vi "Drive Motor TXRX.vi"(0 "Error In":errorcluster, 1 "Drive Motor Handle In":T2, 2 "Open Loop Current Flag":bool, 3 "Tasking Period":dbl, 4 "RPM Control (rad/s)":dbl, 5 "Controller Data In":refnum<data-value>, 6 "Speed Control (m/s)":dbl, 7 "?":T3={"Accelerometer Bias"={"X (m/s)"=0.0, "Y (m/s)"=0.0, "Z (m/s)"=0.0}, "Gyroscope Bias"={"X (m/s)"=0.0, "Y (m/s)"=0.0, "Z (m/s)"=0.0}, "Steering Motor Gear Ratio"=611.0, "Steering Pully Gear Ratio"=1.0, "Steering Encoder CPR"=500.0, "Steering Motor Max RPM"=4000.0, "Wheelbase (m)"=1.12, "Fork Angle (rad)"=1.3, "Balancing Controller"={"Kp (/s)"=0.0, "Kd (1)"=0.0}, "Max Allowed Steering Angle (rad)"=0.7, "Task Periods"={"Emergency Stop (us)"=0, "IMU (us)"=0, "Steering Motor Encoder (us)"=0, "State Estimator (us)"=0, "Balancing Controller (us)"=0, "GNSS (us)"=0, "Logging (us)"=0, "Drive Motor (us)"=0, "Visualization (us)"=50000}, "Drive Motor Gear Ratio"=0.7, "lr"=0.0, "lf"=0.0, "lambda"=0.0, "k1"=0.0, "k2"=0.0, "e1_max"=0.0, "Ad_t"=0.0, "Bd_t"=0.0, "C_t"=0.0, "D_t"=0.0, "Wheel radius"=0.311}, 10 "No Kf":bool, 11 "Ki":dbl, 12 "RPM / Speed":bool, 13 "Kp":dbl, 16 "Open Loop Current":dbl min=0.0, 17 "Kf":dbl min=0.0) -> (14 "Error Out":errorcluster, 15 "Drive Motor Handle Out":T2, 18 "Drive Motor Data":T1, 19 "Controller Data Out":refnum<data-value>)   [LabVIEW 2021]
uses:
  Drive Motor Handle.ctl
  Configuration/Configuration.ctl
  Drive Motor Data.ctl
  Logging/Controller Data.ctl
  Steering Motor/Steering Motor Data.ctl
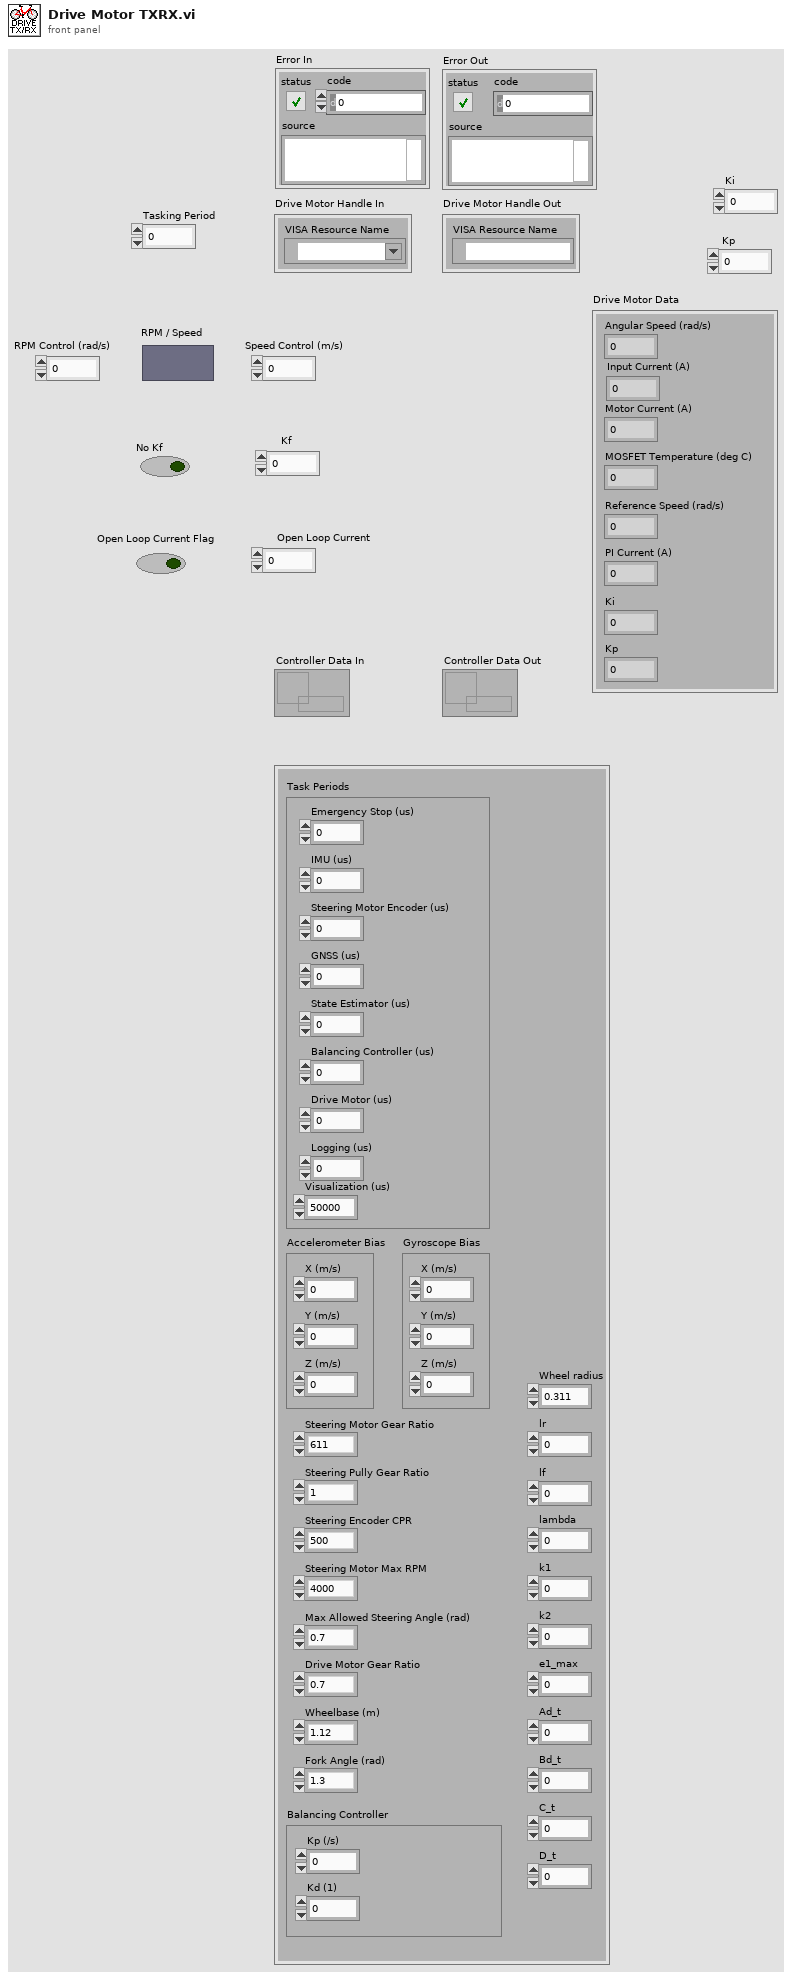
[diagram p1: front panel]
types:
  T1 = typedef "Drive Motor Data.ctl" = cluster{"Angular Speed (rad/s)":dbl, "Input Current (A)":dbl, "Motor Current (A)":dbl, "MOSFET Temperature (deg C)":dbl, "Reference Speed (rad/s)":dbl, "PI Current (A)":dbl, "Ki":dbl, "Kp":dbl}
  T2 = typedef "Drive Motor Handle.ctl" = cluster{"VISA Resource Name":refnum<visa-resource-name>}
  T3 = typedef "Configuration.ctl" = cluster{"Accelerometer Bias":cluster{"X (m/s)":dbl, "Y (m/s)":dbl, "Z (m/s)":dbl}, "Gyroscope Bias":cluster{"X (m/s)":dbl, "Y (m/s)":dbl, "Z (m/s)":dbl}, "Steering Motor Gear Ratio":dbl, "Steering Pully Gear Ratio":dbl, "Steering Encoder CPR":dbl, "Steering Motor Max RPM":dbl, "Wheelbase (m)":dbl, "Fork Angle (rad)":dbl, "Balancing Controller":cluster{"Kp (/s)":dbl, "Kd (1)":dbl}, "Max Allowed Steering Angle (rad)":dbl, "Task Periods":cluster{"Emergency Stop (us)":i64, "IMU (us)":i64, "Steering Motor Encoder (us)":i64, "State Estimator (us)":i64, "Balancing Controller (us)":i64, "GNSS (us)":i64, "Logging (us)":i64, "Drive Motor (us)":i64, "Visualization (us)":i64}, "Drive Motor Gear Ratio":dbl, "lr":dbl, "lf":dbl, "lambda":dbl, "k1":dbl, "k2":dbl, "e1_max":dbl, "Ad_t":dbl, "Bd_t":dbl, "C_t":dbl, "D_t":dbl, "Wheel radius":dbl}
  T4 = typedef "Controller Data.ctl" = cluster{"Drive Motor Data":T1, "Steering Motor Data":T5}
  T5 = typedef "Steering Motor Data.ctl" = cluster{"PWM":dbl, "Steering Angle Rate (rad/s)":dbl, "input balancing":dbl}
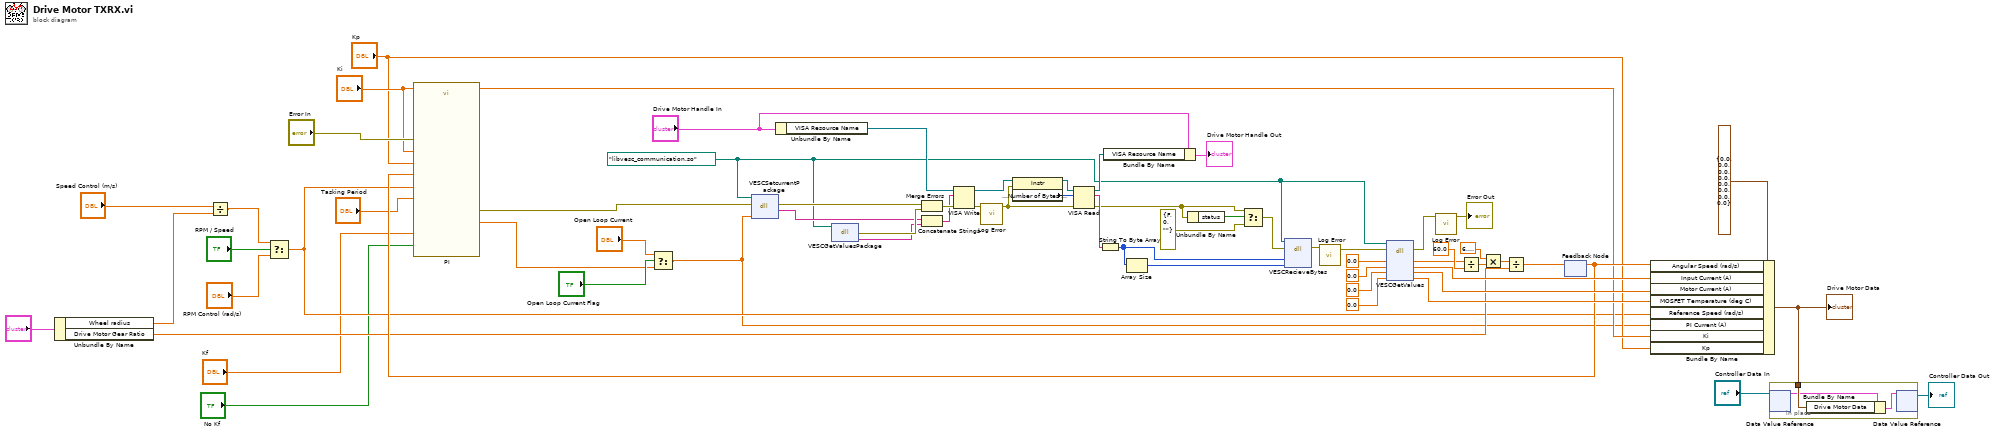
[diagram p0: block diagram]
diagram:
  w21 = path "libvesc_communication.so" ("path in")
  n1 = Unbundle By Name("?") -> ("Wheel radius"=w9:dbl, "Drive Motor Gear Ratio"=w8:dbl)
  n2 = Divide(x="Speed Control (m/s)", y=w9) -> (x/y=w14:dbl)
  n3 = Select(t=w14, s="RPM / Speed", f="RPM Control (rad/s)") -> (s? t:f=w7:dbl)
  n4 = Unbundle By Name("Drive Motor Handle In") -> ("VISA Resource Name"=w60:refnum<visa-resource-name>)
  n5 = dll-call lib="?" fn="VESCGetValuesPackage"(path in=w21) -> (error out=w59:errorcluster, "Package"=w25:string)  [unwired: 2 in, 1 out]
  n6 = feedback #1() -> (w18:dbl)  [unwired: 1 in]
  n7 = call "PI.vi"("Tasking Period"="Tasking Period", "Kp"="Kp", "Reference Speed (rad/s)"=w7, "Ki"="Ki", "Real Speed (rad/s)"=w18, "No Kf"="No Kf", "Kf"="Kf", "Error In"="Error In") -> ("PI Current (A)"=w2:dbl, "Error Out"=w17:errorcluster)  [unwired: 2 in]
  n8 = Select(t="Open Loop Current", s="Open Loop Current Flag", f=w2) -> (s? t:f=w1:dbl)
  n9 = dll-call lib="?" fn="VESCSetcurrentPackage"(path in=w21, error in=w17, "current"=w1) -> (error out=w22:errorcluster, "Package"=w23:string)  [unwired: 2 in, 1 out]
  n10 = Merge Errors(w22, w59) -> (w58:errorcluster)
  n11 = Concatenate Strings(w23, w25) -> (w24:string)
  n12 = VISA Write(VISA resource name=w60, write buffer=w24, error in (no error)=w58) -> (VISA resource name out=w57:refnum<visa-resource-name>, error out=w63:errorcluster)  [unwired: 1 out]
  n13 = call "Log Error.vi"("Error In"=w63) -> ("Error Out"=w45:errorcluster)  [unwired: 10 in]
  n14 = property class="Instr"(reference=w57, error in=w45) -> (reference out=w52:refnum<visa-resource-name>, "Serial Settings:Number of Bytes at Serial Port"=w55:u32)  [unwired: 1 out]
  n15 = VISA Read(VISA resource name=w52, byte count=w55, error in (no error)=w45) -> (VISA resource name out=w56:refnum<visa-resource-name>, read buffer=w54:string, error out=w53:errorcluster)  [unwired: 1 out]
  n16 = String To Byte Array(string=w54) -> (unsigned byte array=w50:u8[])
  n17 = Bundle By Name(cluster="Drive Motor Handle In", "VISA Resource Name"=w56) -> (→"Drive Motor Handle Out":T2)
  n18 = Array Size(array=w50) -> (size(s)=w51:i32)
  n19 = Unbundle By Name(w53) -> ("status"=w49:bool)
  n20 = Select(t=w53, s=w49, f=errorcluster {"status"=FALSE, "code"=0, "source"=""}) -> (s? t:f=w48:errorcluster)
  n21 = dll-call lib="?" fn="VESCRecieveBytes"(path in=w21, error in=w48, "bytes"=w50, "length"=w51) -> (error out=w46:errorcluster)  [unwired: 4 in, 1 out]
  n22 = call "Log Error.vi"("Error In"=w46) -> ("Error Out"=w26:errorcluster)  [unwired: 10 in]
  n23 = dll-call lib="?" fn="VESCGetValues"(path in=w21, error in=w26, "RPM"=0.0, "currentIn"=0.0, "currentMotor"=0.0 ("RPM"), "tempMOS"=0.0 ("currentIn")) -> (error out=w36:errorcluster, "RPM"=w34:dbl, "currentIn"=w33:dbl, "currentMotor"=w38:dbl, "tempMOS"=w27:dbl)  [unwired: 2 in, 1 out]
  n24 = call "Log Error.vi"("Error In"=w36) -> ("Error Out"=→"Error Out":errorcluster)  [unwired: 10 in]
  n25 = Divide(x=w34, y=60.0 ("x")) -> (x/y=w40:dbl)
  n26 = Multiply(x=6.283185307179586, y=w40) -> (x*y=w32:dbl)
  n27 = Divide(x=w32, y=w8) -> (x/y=w19:dbl)
  n28 = feedback-in #1(w19) -> ()
  n29 = Bundle By Name(cluster=T1 {"Angular Speed (rad/s)"=0.0, "Input Current (A)"=0.0, "Motor Current (A)"=0.0, "MOSFET Temperature (deg C)"=0.0, "Reference Speed (rad/s)"=0.0, "PI Current (A)"=0.0, "Ki"=0.0, "Kp"=0.0} ("Drive Motor Data"), "Angular Speed (rad/s)"=w18, "Input Current (A)"=w33, "Motor Current (A)"=w38, "MOSFET Temperature (deg C)"=w27, "Reference Speed (rad/s)"=w7, "PI Current (A)"=w1, "Ki"="Ki", "Kp"="Kp") -> (w29:T1)
  "Drive Motor Data" <- w29
  n30 = in-place {
    in-place-border: w29 -> [w66]
    n31 = in-place-dvr #2("Controller Data In") -> (w65:T4)  [unwired: 1 out]
    n32 = Bundle By Name(cluster=w65, "Drive Motor Data"=w66) -> (w67:T4)
    n33 = in-place-dvr #2(w67) -> (→"Controller Data Out":refnum<data-value>)  [unwired: 1 out]
  }
